vi "check_5181.vi"() -> ()   [LabVIEW 2013]
panel:
  in  "R&S address":string="29"
  out "address 2":string
  in  "amplitude (mV)":i32=10
  in  "modulation (kHz)":i32=100
  in  "center frequency (MHz)":dbl=32.7
  in  "exit":bool
  in  "rs_set":bool
  in  "rs_off":bool
  in  "rs_on":bool
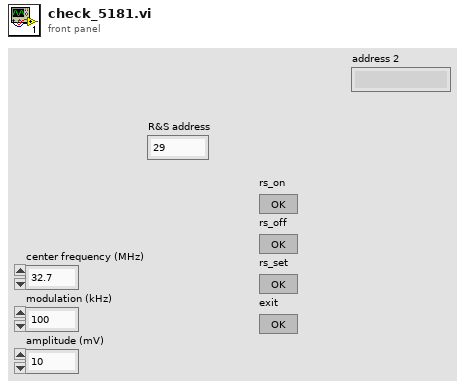
[diagram p1: front panel]
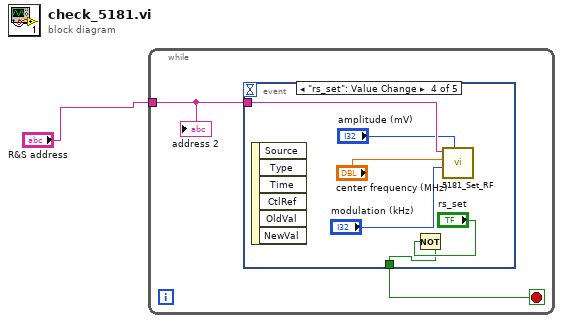
[diagram p0: block diagram]
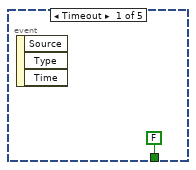
[diagram p2: hidden frame]
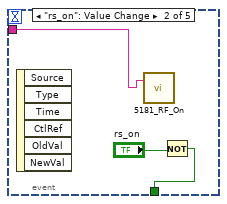
[diagram p3: hidden frame]
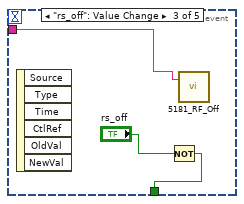
[diagram p4: hidden frame]
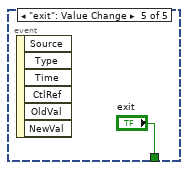
[diagram p5: hidden frame]
diagram:
  n1 = while {
    tunnel: "R&S address" -> [w2]
    stop <- w3 stop-if-true
    n2 = event shown="[3] \"rs_set\": Value Change" {
      selector: _ -> [_ _ _ _ _]
      dyn-events: _ -> [_ _ _ _ _]
      timeout: _ -> [_ _ _ _ _]
      tunnel: [FALSE ("exit") w6 w9 w15 "exit"] -> w3
      tunnel: w2 -> [_ w5 w8 w14 _]
      event Timeout {
        n3 = event-data() -> ()  [unwired: 1 in, 3 out]
      }
      event "rs_on": Value Change {
        n4 = event-data() -> ()  [unwired: 1 in, 6 out]
        n5 = call "5181_RF_On.vi"("address"=w5) -> ()  [unwired: 1 in, 2 out]
        n6 = Not(x="rs_on") -> (.not. x?=w6:bool)
      }
      event "rs_off": Value Change {
        n7 = event-data() -> ()  [unwired: 1 in, 6 out]
        n8 = Not(x="rs_off") -> (.not. x?=w9:bool)
        n9 = call "5181_RF_Off.vi"("address"=w8) -> ()  [unwired: 1 in, 2 out]
      }
      event "rs_set": Value Change {
        n10 = event-data() -> ()  [unwired: 1 in, 6 out]
        n11 = Not(x="rs_set") -> (.not. x?=w15:bool)
        n12 = call "5181_Set_RF.vi"("address"=w14, "center frequency (MHz)"="center frequency (MHz)", "modulation (kHz)"="modulation (kHz)", "amplitude (mV)"="amplitude (mV)") -> ()  [unwired: 1 in, 2 out]
      }
      event "exit": Value Change {
        n13 = event-data() -> ()  [unwired: 1 in, 6 out]
      }
    }
    "address 2" <- w2
  }
